vi "6b - State Machine Basics.vi"() -> ()   [LabVIEW 2010]
doc: "Exercise 1.3\nThis VI uses the Cluster to Array function to convert an array of Boolean values into an array of Boolean values. This is a very convenient way to build user interface VIs for menuing systems.\n\nThe VI searches the array of Boolean values for a TRUE value, which indicates that the user pressed a button. Based on this value, the VI uses a Case Structure to execute code. You will expand this VI in future exercises to actually implement the menu options.\n\nYou will use this VI as the basis for Application Exercise.vi (Exercise 6.1), in which you combine several of the VIs you create in this course into a larger project."
panel:
  in  "Message":string
  in  "menu cluster":T1
  # "This problem is same as the previous one (1b - cluster) but the\ndiagram is somewhat different. It employs a shift register. Note \nthat after executing your action it returns to no event (i.e. no button\npressed case so that the VI begins monitoring the buttons on the\nfront panel as soon as possible."
  # "Mechanical Action: Latch When Released"
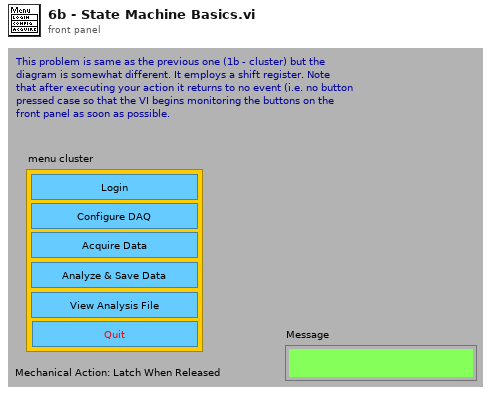
[diagram p1: front panel]
types:
  T1 = cluster{"Login":bool, "Configure Data Acquisition":bool, "Acquire Data":bool, "Analyze & Present Data":bool, "View":bool, "Quit":bool}
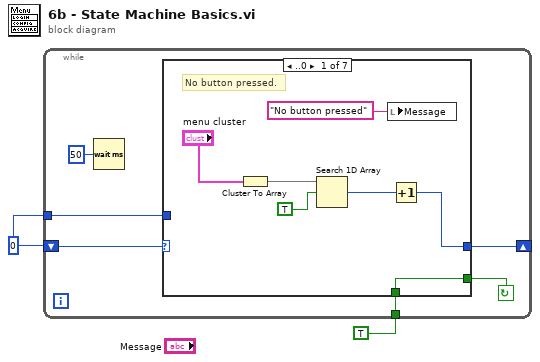
[diagram p0: block diagram]
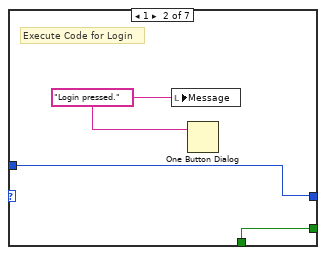
[diagram p2: hidden frame]
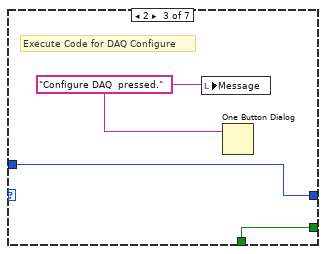
[diagram p3: hidden frame]
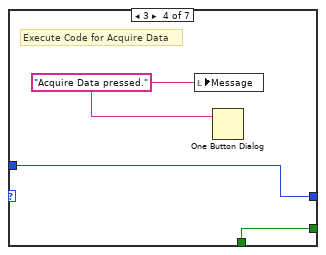
[diagram p4: hidden frame]
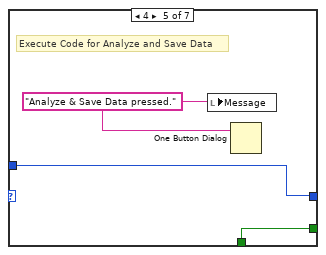
[diagram p5: hidden frame]
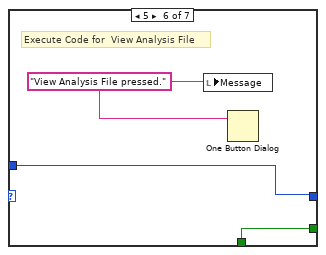
[diagram p6: hidden frame]
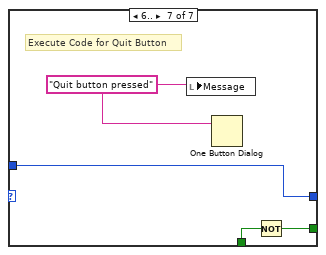
[diagram p7: hidden frame]
diagram:
  w2 = 0
  n1 = while {
    tunnel: w2 -> [w3]
    tunnel: TRUE ("Continue") -> [w5]
    shift-left: w2 -> [w8]
    shift-right: [w7] -> _
    stop <- w4 continue-if-true
    n2 = Wait (ms)(milliseconds to wait=u32 50) -> ()  [unwired: 1 out]
    n3 = case shown="..0" w8 {
      tunnel: [w11 w17 w20 w23 w26 w29 w34] -> w7
      tunnel: w5 -> [w10 w18 w21 w24 w27 w30 w33]
      tunnel: [w10 w18 w21 w24 w27 w30 w32] -> w4
      tunnel: w3 -> [_ w17 w20 w23 w26 w29 w34]
      frame ..0 {
        # "No button pressed."
        n4 = Cluster To Array(cluster="menu cluster") -> (array=w15:bool[])
        n5 = Search 1D Array(1D array=w15, element=TRUE) -> (index of element=w13:i32)  [unwired: 1 in]
        n6 = local write "Message"("No button pressed" ("Message")) -> ()
        n7 = Increment(x=w13) -> (x+1=w11:i32)
      }
      frame 1 {
        w16 = "Login pressed."
        # "Execute Code for Login"
        n8 = local write "Message"(w16) -> ()
        n9 = One Button Dialog(message=w16) -> ()  [unwired: 1 in, 1 out]
      }
      frame 2 {
        w19 = "Configure DAQ  pressed."
        # "Execute Code for DAQ Configure"
        n10 = local write "Message"(w19) -> ()
        n11 = One Button Dialog(message=w19) -> ()  [unwired: 1 in, 1 out]
      }
      frame 3 {
        w22 = "Acquire Data pressed."
        # "Execute Code for Acquire Data"
        n12 = local write "Message"(w22) -> ()
        n13 = One Button Dialog(message=w22) -> ()  [unwired: 1 in, 1 out]
      }
      frame 4 {
        w25 = "Analyze & Save Data pressed."
        # "Execute Code for Analyze and Save Data"
        n14 = local write "Message"(w25) -> ()
        n15 = One Button Dialog(message=w25) -> ()  [unwired: 1 in, 1 out]
      }
      frame 5 {
        w28 = "View Analysis File pressed."
        # "Execute Code for  View Analysis File"
        n16 = local write "Message"(w28) -> ()
        n17 = One Button Dialog(message=w28) -> ()  [unwired: 1 in, 1 out]
      }
      frame 6.. {
        w31 = "Quit button pressed" ("message")
        # "Execute Code for Quit Button"
        n18 = local write "Message"(w31) -> ()
        n19 = One Button Dialog(message=w31) -> ()  [unwired: 1 in, 1 out]
        n20 = Not(x=w33) -> (.not. x?=w32:bool)
      }
    }
  }
